vi "Post-Install Custom Action.vi"(10 "Variant":variant) -> (0 "error out":errorcluster)   [LabVIEW 2019]
uses:
  <vilib>/Utility/traverseref.llb/TRef TravTarget.ctl
  <vilib>/Utility/traverseref.llb/VI Scripting - Traverse.lvlib
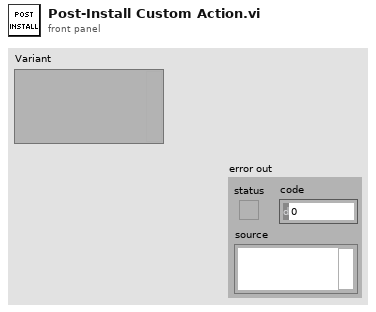
[diagram p1: front panel]
types:
  T1 = typedef "TRef TravTarget.ctl" = enum16{"FP", "BD", "Other"}
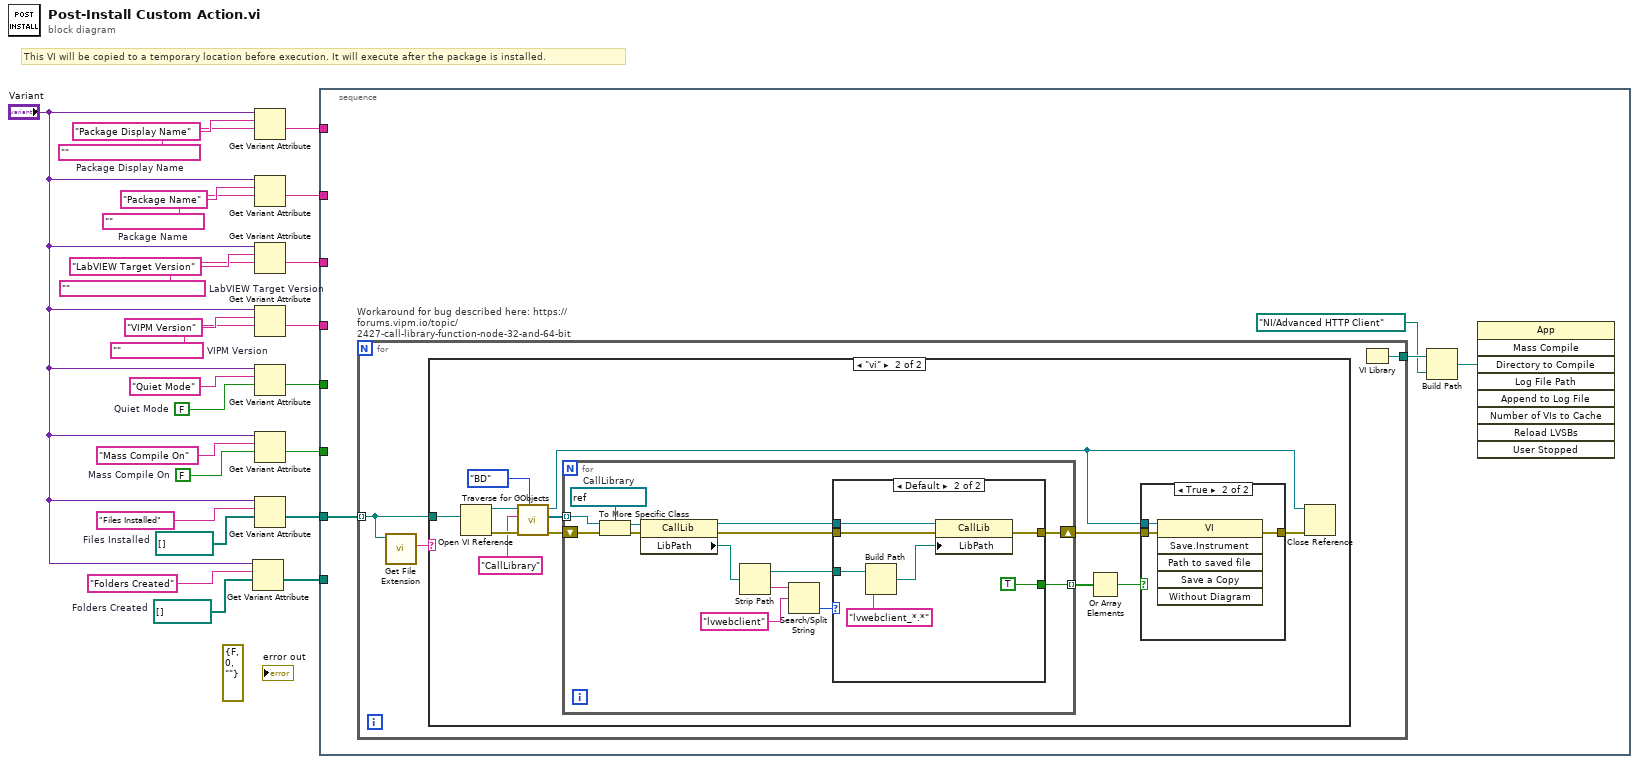
[diagram p0: block diagram]
diagram:
  (unwired) errorcluster {"status"=FALSE, "code"=0, "source"=""} ("error out")
  w1 = path[] []  # Folders Created
  w2 = path[] []  # Files Installed
  w8 = FALSE  # Mass Compile On
  w9 = ""  # Package Display Name
  w16 = FALSE  # Quiet Mode
  w19 = ""  # VIPM Version
  w21 = ""  # LabVIEW Target Version
  w23 = ""  # Package Name
  # "This VI will be copied to a temporary location before execution. It will execute after the package is installed."
  n1 = Get Variant Attribute(Variant="Variant", name="Folders Created", default value (empty Variant)=w1) -> (value=w6:path[])  [unwired: 1 in, 3 out]
  n2 = Get Variant Attribute(Variant="Variant", name="Package Display Name", default value (empty Variant)=w9) -> (value=w15:string)  [unwired: 1 in, 3 out]
  n3 = Get Variant Attribute(Variant="Variant", name="Package Name", default value (empty Variant)=w23) -> (value=w14:string)  [unwired: 1 in, 3 out]
  n4 = Get Variant Attribute(Variant="Variant", name="LabVIEW Target Version", default value (empty Variant)=w21) -> (value=w13:string)  [unwired: 1 in, 3 out]
  n5 = Get Variant Attribute(Variant="Variant", name="VIPM Version", default value (empty Variant)=w19) -> (value=w12:string)  [unwired: 1 in, 3 out]
  n6 = Get Variant Attribute(Variant="Variant", name="Quiet Mode", default value (empty Variant)=w16) -> (value=w11:bool)  [unwired: 1 in, 3 out]
  n7 = Get Variant Attribute(Variant="Variant", name="Mass Compile On", default value (empty Variant)=w8) -> (value=w10:bool)  [unwired: 1 in, 3 out]
  n8 = Get Variant Attribute(Variant="Variant", name="Files Installed", default value (empty Variant)=w2) -> (value=w5:path[])  [unwired: 1 in, 3 out]
  n9 = stacked-sequence {
    tunnel: w15 -> [_]
    tunnel: w14 -> [_]
    tunnel: w13 -> [_]
    tunnel: w12 -> [_]
    tunnel: w11 -> [_]
    tunnel: w10 -> [_]
    tunnel: w5 -> [w28]
    tunnel: w6 -> [_]
    frame #0 {
      n10 = for "Workaround for bug described here: https://forums.vipm.io/topic/2427-call-library-function-node-32-and-64-bit" {
        tunnel: w28 -> [w32] mode=indexing
        tunnel: [w31] -> w27
        n11 = call <vilib>:"Get File Extension.vi"("file"=w32) -> ("lowercase file extension"=w30:string)  [unwired: 6 in, 4 out]
        n12 = case shown="\"vi\"" w30 {
          tunnel: w32 -> [_ w44]
          frame "False", Default {
          }
          frame "vi" {
            n13 = Open VI Reference(vi path=w44) -> (vi reference=w42:refnum<vi>, error out=w43:errorcluster)  [unwired: 5 in]
            n14 = call <vilib>:"Traverse for GObjects.vi"("Traverse Target"=TRef_TravTarget."BD", "error in (no error)"=w43, "Class Name"="CallLibrary", "VI Refnum"=w42) -> ("error out"=w38:errorcluster, "References"=w39:refnum<vi>[], "dup VI Refnum"=w35:refnum<vi>)  [unwired: 4 in, 1 out]
            n15 = for {
              tunnel: w39 -> [w61] mode=indexing
              shift-right: [w52] -> w37
              shift-left: w38 -> [w62]
              tunnel: [w49] -> w34 mode=indexing
              w60 = refnum<vi> refnum  # CallLibrary
              n16 = To More Specific Class(target class=w60, reference=w61, error in=w62) -> (specific class reference=w58:refnum<vi>, error out=w59:errorcluster)
              n17 = property class="CallLib"(reference=w58, error in=w59) -> (reference out=w53:refnum<vi>, error out=w54:errorcluster, "LibPath"=w57:path)
              n18 = Strip Path(path=w57) -> (stripped path=w50:path, name=w56:string)
              n19 = Search/Split String(string=w56, search string/char (-)="lvwebclient") -> (offset of match=w51:i32)  [unwired: 1 in, 2 out]
              n20 = case shown="Default" w51 {
                tunnel: w54 -> [w63 w70]
                tunnel: w53 -> [_ w69]
                tunnel: [w63 w68] -> w52
                tunnel: w50 -> [_ w67]
                tunnel: [_ TRUE] -> w49
                frame -1 {
                }
                frame Default {
                  n21 = Build Path(base path=w67, name or relative path="lvwebclient_*.*") -> (appended path=w66:path)
                  n22 = property class="CallLib"(reference=w69, error in=w70, "LibPath"=w66) -> (error out=w68:errorcluster)  [unwired: 1 out]
                }
              }
            }
            n23 = Or Array Elements(Boolean array=w34) -> (logical OR=w33:bool)
            n24 = case shown="True" w33 {
              tunnel: w37 -> [w45 w48]
              tunnel: w35 -> [_ w47]
              tunnel: [w45 w46] -> w36
              frame False {
              }
              frame True {
                n25 = invoke class="VI" method="Save.Instrument"(reference=w47, error in=w48) -> (error out=w46:errorcluster)  [unwired: 4 in, 5 out]
              }
            }
            n26 = Close Reference(reference=w35, error in (no error)=w36) -> ()  [unwired: 1 out]
          }
        }
        n27 = VI Library() -> (path=w31:path)
      }
      n28 = Build Path(base path=w27, name or relative path=path "NI/Advanced HTTP Client") -> (appended path=w29:path)
      n29 = invoke class="App" method="Mass Compile"("Directory to Compile"=w29) -> ()  [unwired: 8 in, 9 out]
    }
  }
